vi "compressor rig file save headerline.vi"(11 "fileIO":T1) -> (3 "compressorRig save file headerline":string)   [LabVIEW 2018]
uses:
  type defs/file IO data.ctl
  type defs/channelControl.ctl
  RT/Type Defs/channelScalingTypes.ctl
  RT/Type Defs/scalingMethods.ctl
  Github/ICL-LabVIEW_General/data channels/parent class/Data Channel.lvclass
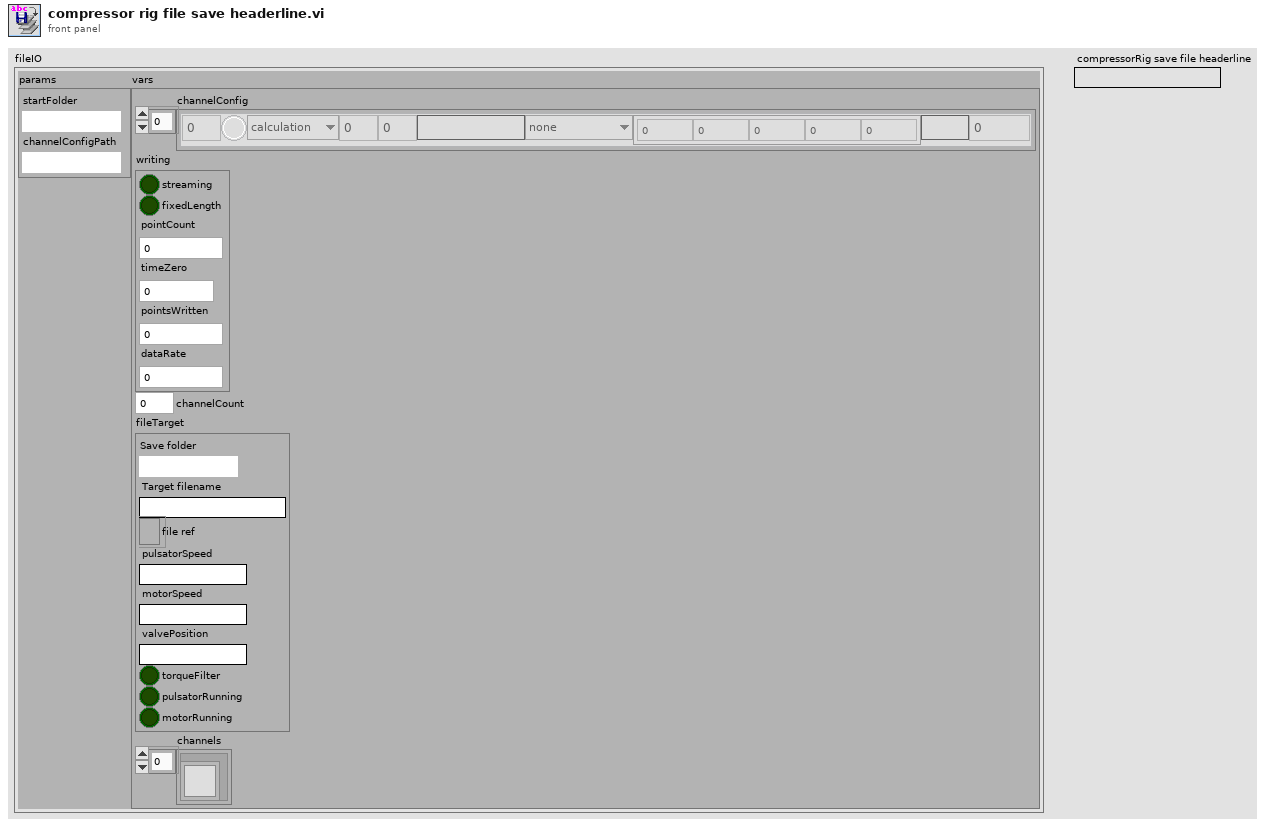
[diagram p1: front panel]
types:
  T1 = typedef "file IO data.ctl" = cluster{"params":cluster{"startFolder":path, "channelConfigPath":path}, "vars":cluster{"channelConfig ":T2[], "writing":cluster{"streaming":bool, "fixedLength":bool, "pointCount":u32, "timeZero":dbl, "pointsWritten":u32, "dataRate":u16}, "channelCount":u16, "fileTarget":cluster{"Save folder":path, "Target filename":string, "file ref":refnum<file>, "pulsatorSpeed":string, "motorSpeed":string, "valvePosition":string, "torqueFilter":bool, "pulsatorRunning":bool, "motorRunning":bool}, "channels":refnum<class "Data Channel.lvclass">[]}}
  T2 = typedef "channelControl.ctl" = cluster{"index":u16, "active":bool, "channelType":T3, "module":u16, "terminal":u16, "channelName":string, "scalingMethod":T4, "scalingParameters":dbl[], "scaledUnits":string, "tempOffset":dbl}
  T3 = typedef "channelScalingTypes.ctl" = enum16{"calculation", "measurement", "scanivalve", "output", "digital"}
  T4 = typedef "scalingMethods.ctl" = enum16{"none", "linear", "thermocouple", "polynomial", "encoder", "RTD"}
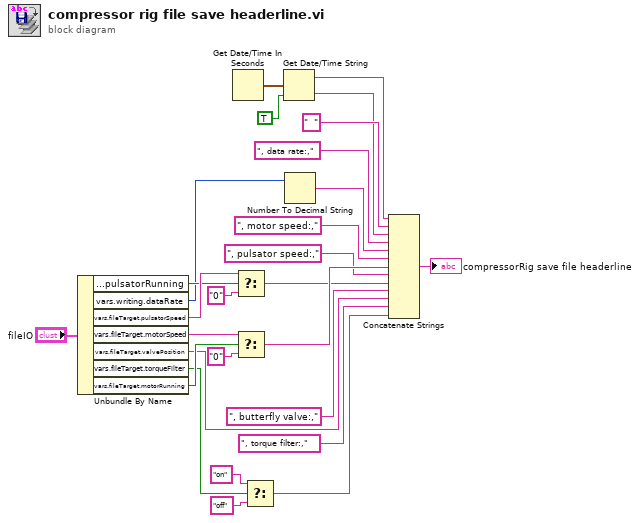
[diagram p0: block diagram]
diagram:
  n1 = Unbundle By Name("fileIO") -> ("vars.fileTarget.pulsatorRunning"=w20:bool, "vars.writing.dataRate"=w10:u16, "vars.fileTarget.pulsatorSpeed"=w21:string, "vars.fileTarget.motorSpeed"=w25:string, "vars.fileTarget.valvePosition"=w14:string, "vars.fileTarget.torqueFilter"=w16:bool, "vars.fileTarget.motorRunning"=w26:bool)
  n2 = Get Date/Time In Seconds() -> (seconds since 1Jan1904=w2:timestamp)
  n3 = Select(t=w21, s=w20, f="0") -> (s? t:f=w23:string)
  n4 = Select(t=w25, s=w26, f="0") -> (s? t:f=w27:string)
  n5 = Select(t="on" ("string"), s=w16, f="off" ("string")) -> (s? t:f=w19:string)
  n6 = Get Date/Time String(seconds (now)=w2, want seconds? (F)=TRUE) -> (date string=w3:string, time string=w4:string)  [unwired: 1 in]
  n7 = Number To Decimal String(number=w10) -> (decimal integer string=w8:string)  [unwired: 1 in]
  n8 = Concatenate Strings(w3, "  " ("string"), w4, ", data rate:," ("string"), w8, ", motor speed:," ("string"), w27, ", pulsator speed:," ("string"), w23, ", butterfly valve:," ("string"), w14, ", torque filter:," ("string"), w19) -> (→"compressorRig save file headerline":string)
